vi "readSelectedCategory.vi"(8 "error in (no error)":errorcluster, 11 "CategoryListUIAdapter in":refnum<class "CategoryListUIAdapter.lvclass">) -> (0 "error out":errorcluster, 2 "Category.lvclass":refnum<class "Category.lvclass">, 3 "CategoryListUIAdapter out":refnum<class "CategoryListUIAdapter.lvclass">)   [LabVIEW 2018, in "CategoryListUIAdapter.lvclass"]
uses:
  CategoryListUIAdapter.lvclass
  Category/Category.lvclass
  <vilib>/Utility/miscctls.llb/LVRowAndColumnTypeDef.ctl
  CategoryListUIAdapter.lvclass/CategoryListUIAdapter.ctl
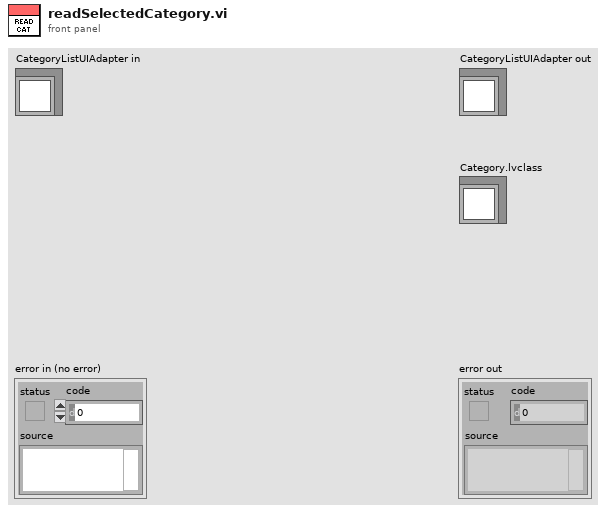
[diagram p1: front panel]
types:
  T1 = typedef "LVRowAndColumnTypeDef.ctl" = cluster{"Row":i32, "Column":i32}
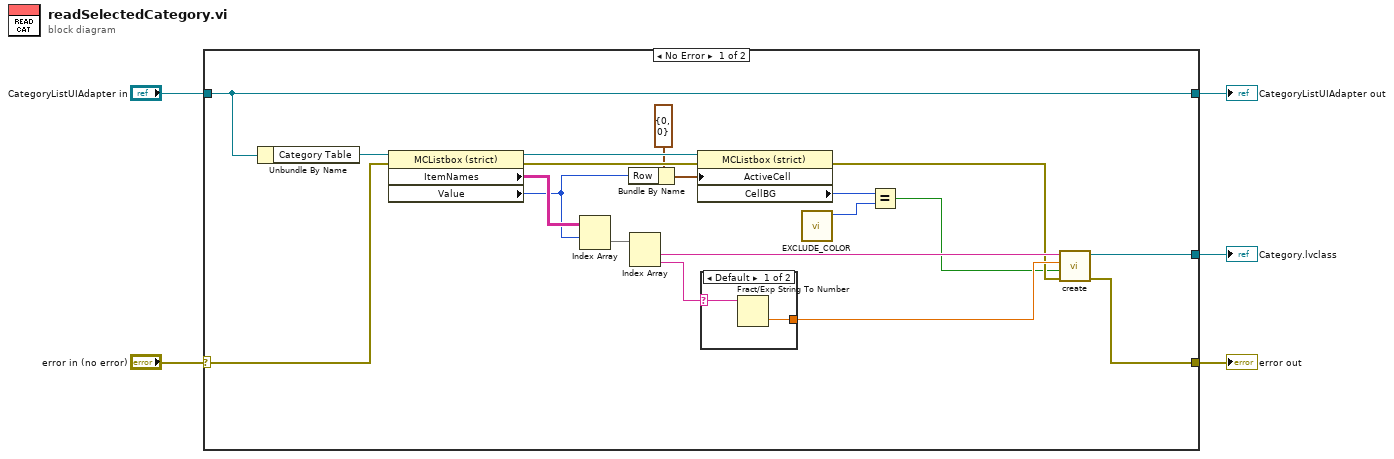
[diagram p0: block diagram]
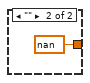
[diagram p2: hidden frame]
diagram:
  n1 = case shown="No Error" "error in (no error)" {
    selector: "error in (no error)" -> [w18 w29]
    tunnel: [w17 w29] -> w4
    tunnel: [w20 w28] -> w2
    tunnel: "CategoryListUIAdapter in" -> [w20 w28]
    tunnel: [w15 _] -> w1
    frame No Error {
      n2 = Unbundle By Name(w20) -> ("Category Table"=w19:refnum<vi>)
      n3 = property class="MCListbox (strict)"(reference=w19, error in=w18) -> (reference out=w14:refnum<vi>, error out=w13:errorcluster, "ItemNames"=w16:string[][], "Value"=w9:i32)
      n4 = Index Array(array=w16, index (row)=w9) -> (element=w24:string[])  [unwired: 1 in]
      n5 = Bundle By Name(cluster=T1 {"Row"=0, "Column"=0} ("Active Cell:Active Cell"), "Row"=w9) -> (w10:T1)
      n6 = Index Array(array=w24) -> (element #1=w23:string, element #2=w22:string)  [unwired: 2 in]
      n7 = property class="MCListbox (strict)"(reference=w14, error in=w13, "ActiveCell"=w10) -> (error out=w12:errorcluster, "CellBG"=w8:u32)  [unwired: 1 out]
      n8 = case shown="Default" w22 {
        selector: w22 -> [w26 _]
        tunnel: [w25 nan] -> w21
        frame Default {
          n9 = Fract/Exp String To Number(string=w26) -> (number=w25:dbl)  [unwired: 3 in, 1 out]
        }
        frame "" {
        }
      }
      n10 = call "EXCLUDE_COLOR.vi"() -> ("Color Box"=w7:u32)  [unwired: 11 in]
      n11 = Equal?(x=w8, y=w7) -> (x = y?=w6:bool)
      n12 = call "create.vi"("error in (no error)"=w12, "DefaultExclude"=w6, "Default Goal Amount"=w21, "Name"=w23) -> ("error out"=w17:errorcluster, "Category out"=w15:refnum<class "Category.lvclass">)  [unwired: 6 in]
    }
    frame Error {
    }
  }
  "error out" <- w4
  "CategoryListUIAdapter out" <- w2
  "Category.lvclass" <- w1
